vi "Read DAQmx Task.vi"(8 "error in (no error)":errorcluster, 11 "DAQmx Actor in":refnum<class "DAQmx Actor.lvclass">) -> (0 "error out":errorcluster, 2 "DAQmx Task":refnum<k21>, 3 "DAQmx Actor out":refnum<class "DAQmx Actor.lvclass">)   [LabVIEW 2024, in "DAQmx Actor.lvlib" / "DAQmx Actor.lvclass"]
uses:
  DAQmx Actor.lvclass
  DAQmx Actor.lvclass/DAQmx Actor.ctl
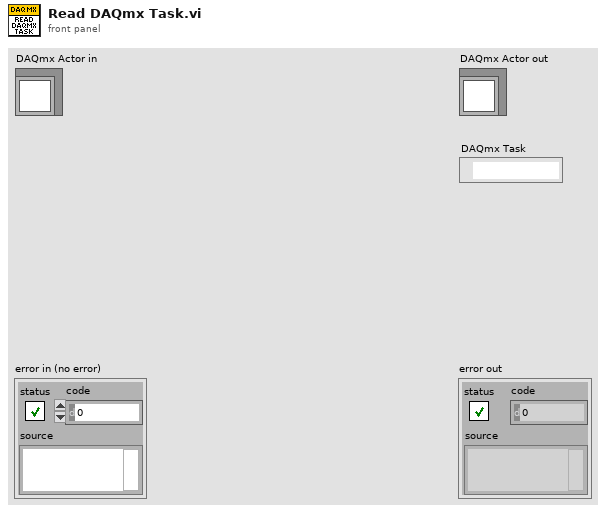
[diagram p1: front panel]
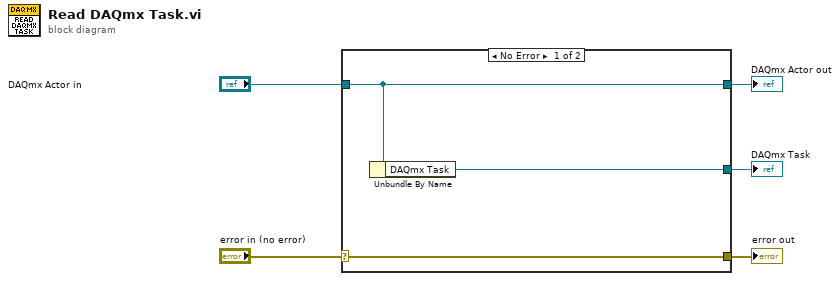
[diagram p0: block diagram]
diagram:
  n1 = case shown="No Error" "error in (no error)" {
    selector: "error in (no error)" -> [w8 w9]
    tunnel: [w8 w9] -> w4
    tunnel: [w7 w10] -> w2
    tunnel: "DAQmx Actor in" -> [w7 w10]
    tunnel: [w6 _] -> w1
    frame No Error {
      n2 = Unbundle By Name(w7) -> ("DAQmx Task"=w6:refnum<k21>)
    }
    frame Error {
    }
  }
  "error out" <- w4
  "DAQmx Actor out" <- w2
  "DAQmx Task" <- w1
